vi "TDMSGetSelectedData.vi"(11 "TraceName":string="D:\\Vi\\Data\\Singapore\\170620\\data_145.tdms: 3") -> (1 "F (pN)":dbl[](array[numeric]), 2 "Z (um)":dbl[](array[numeric]), 3 "Time (s)":dbl[](array[numeric]))   [LabVIEW 2018]
panel:
  out "Waveform Graph 2":dbl[](graph)
  out "Waveform Graph":dbl[][](graph)
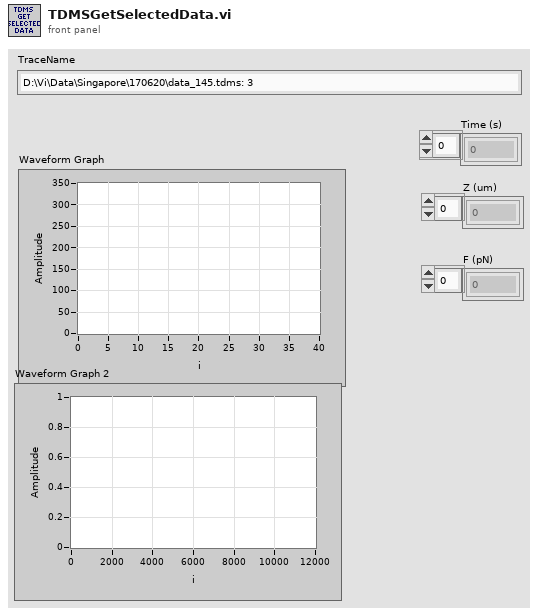
[diagram p1: front panel]
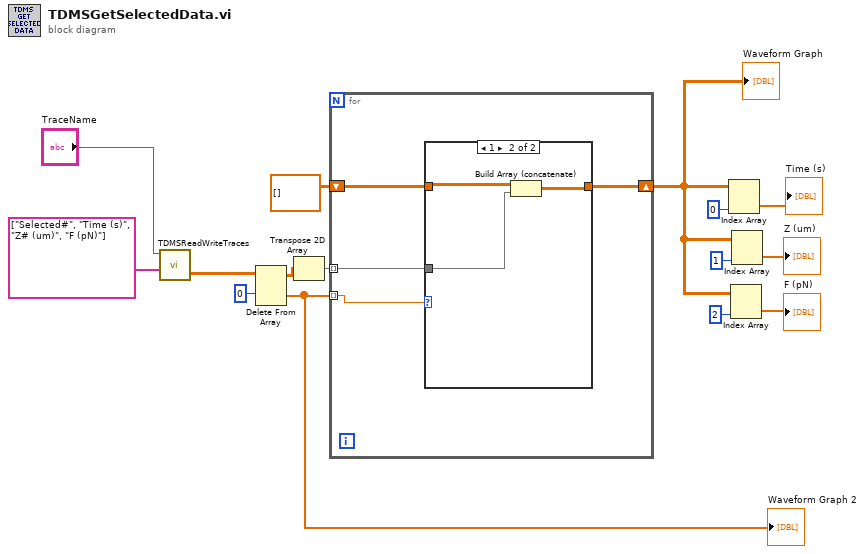
[diagram p0: block diagram]
diagram:
  n1 = call "TDMSReadWriteTraces.vi"("Channels in"=string[] ["Selected#", "Time (s)", "Z# (um)", "F (pN)"] ("channel name(s) in"), "tracename"="TraceName") -> ("Data out"=w13:dbl[][])  [unwired: 4 in, 5 out]
  n2 = Delete From Array(array=w13, index (row)=0) -> (deleted portion=w1:dbl[], array with subset deleted=w11:dbl[][])  [unwired: 2 in]
  "Waveform Graph 2" <- w1
  n3 = Transpose 2D Array(2D array=w11) -> (transposed array=w10:dbl[][])
  n4 = for {
    tunnel: w1 -> [w19] mode=indexing
    shift-right: [w18] -> w2
    shift-left: dbl[][] [] -> [w17]
    tunnel: w10 -> [w16] mode=indexing
    n5 = case shown="1" w19 {
      tunnel: [w20 w21] -> w18
      tunnel: w17 -> [w20 w23]
      tunnel: w16 -> [_ w22]
      frame 0, Default {
      }
      frame 1 {
        n6 = Build Array (concatenate)(w23, w22) -> (w21:dbl[][])
      }
    }
  }
  "Waveform Graph" <- w2
  n7 = Index Array(array=w2, index (col)=0 ("disabled index (col)")) -> (element=→"Time (s)":dbl[])  [unwired: 1 in]
  n8 = Index Array(array=w2, index (col)=2 ("disabled index (col)")) -> (element=→"F (pN)":dbl[])  [unwired: 1 in]
  n9 = Index Array(array=w2, index (col)=1 ("disabled index (col)")) -> (element=→"Z (um)":dbl[])  [unwired: 1 in]
